vi "_Raise Notification Received.vi"(4 "WebView2.lvlib:WebView2 Control.lvclass":refnum<class "WebView2 Control.lvclass">, 5 "Event Data":cluster{"sender":refnum<k24>, "e":refnum<k24>}, 6 "Control Ref":refnum<k24>, 7 "Event Common Data":T1) -> ()   [LabVIEW 2025, in "WebView2.lvlib" / "WebView2 Control.lvclass"]
uses:
  WebView2 Control.lvclass
  WebView2 Control.lvclass/WebView2 Control.ctl
  E:/Labview/LV 2023/PPL/PPL Builder/Libs/LV-WebView2/Source/Libs/Microsoft.Web.WebView2.Core.dll
  Libs/Microsoft.Web.WebView2.Core.dll
  Notification Received Event Data.ctl
  WebView2 Event Filter Interface/WebView2 Event Filter Interface.lvclass
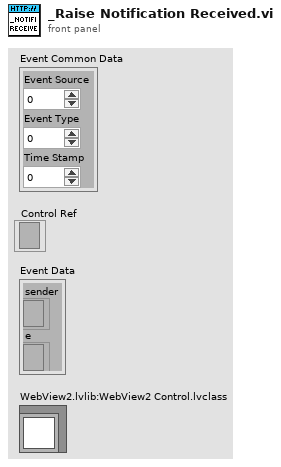
[diagram p1: front panel]
types:
  T1 = cluster{"Event Source":i32, "Event Type":u32, "Time Stamp":u32}
  T2 = typedef "WebView2.lvlib/WebView2 Control.lvclass/Notification Received Event Data.ctl" = cluster{"Notification":refnum<k24>, "SenderOrigin":string}
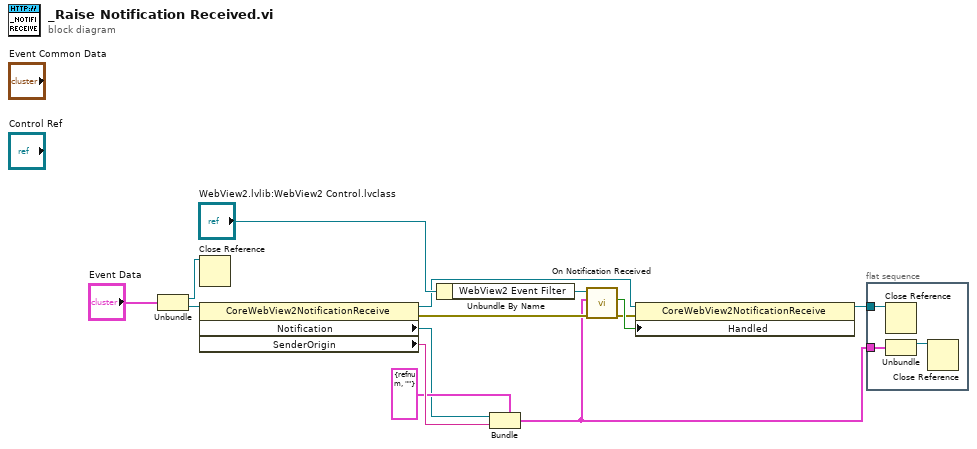
[diagram p0: block diagram]
diagram:
  n1 = Unbundle("Event Data") -> ("sender"=w13:refnum<k24>, "e"=w12:refnum<k24>)
  n2 = Close Reference(reference=w13) -> ()  [unwired: 1 in, 1 out]
  n3 = property class="CoreWebView2NotificationReceive"(reference=w12) -> (reference out=w6:refnum<k24>, error out=w7:errorcluster, "Notification"=w2:refnum<k24>, "SenderOrigin"=w11:string)  [unwired: 1 in]
  n4 = Unbundle By Name("WebView2.lvlib:WebView2 Control.lvclass") -> ("WebView2 Event Filter"=w8:refnum<class "WebView2 Event Filter Interface.lvclass">)
  n5 = Bundle(cluster=T2 {"Notification"=refnum, "SenderOrigin"=""}, "Notification"=w2, "SenderOrigin"=w11) -> (w1:T2)
  n6 = call-dynamic "On Notification Received.vi"("error in (no error)"=w7, "Data"=w1, "WebView2 Event Filter Interface in"=w8) -> ("error out"=w4:errorcluster, "Handled"=w5:bool)  [unwired: 7 in]
  n7 = property class="CoreWebView2NotificationReceive"(reference=w6, error in=w4, "Handled"=w5) -> (reference out=w3:refnum<k24>)  [unwired: 1 out]
  n8 = flat-sequence {
    tunnel: w3 -> [w17]
    tunnel: w1 -> [w16]
    frame #0 {
      n9 = Close Reference(reference=w17) -> ()  [unwired: 1 in, 1 out]
      n10 = Unbundle(w16) -> ("Notification"=w15:refnum<k24>)  [unwired: 1 out]
      n11 = Close Reference(reference=w15) -> ()  [unwired: 1 in, 1 out]
    }
  }
